vi "UDCLogMessage.vi"(8 "Error In":errorcluster, 10 "value":string, 11 "name":string) -> (0 "Error Out":errorcluster)   [LabVIEW 2020, in "niceiplib.lvlib"]
doc: "This is the API that logs the message in the form of Key, Value pairs. This is adepreciated API and must not be used unless there is an specific requirement.\n\nIn all other cases UDCLogUsageData.vi must be used."
uses:
  <vilib>/UDC/niceiplib.lvlib
panel:
  # "@param[in]\tname\t\t\t\tName of the data being logged\n @param[in]\tvalue\t\t\t\tValue of the data being logged."
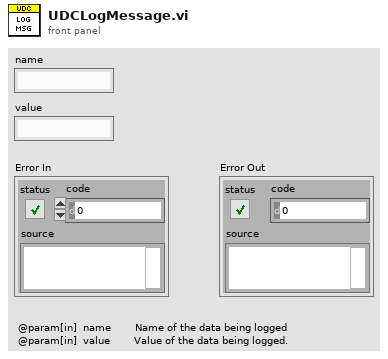
[diagram p1: front panel]
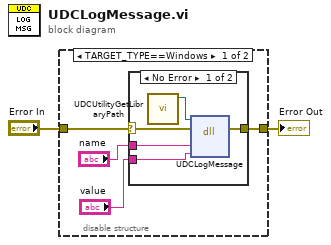
[diagram p0: block diagram]
diagram:
  n1 = disable-structure shown="TARGET_TYPE==Windows" {
    disable-tunnel: [w4 w13] -> w2
    disable-tunnel: "Error In" -> [w3 w13]
    frame condition #0 (active) {
      n2 = case shown="No Error" w3 {
        selector: w3 -> [w8 w12]
        tunnel: "name" -> [w11 _]
        tunnel: "value" -> [w10 _]
        tunnel: [w9 w12] -> w4
        frame No Error {
          n3 = call <vilib>:"UDCUtilityGetLibraryPath.vi"() -> ("Library Path"=w7:path)  [unwired: 11 in]
          n4 = dll-call lib="C:/2013LabVIEWCode/dist/vi.lib/UDC/niceiplib.*" fn="UDCLogMessage"(path in=w7, error in=w8, "name"=w11, "value"=w10) -> (error out=w9:errorcluster)  [unwired: 4 in, 1 out]
        }
        frame Error {
        }
      }
    }
    frame condition #1 {
    }
  }
  "Error Out" <- w2
